vi "4155C Config VAR2 params.vi"(4 "power compliance (0 = OFF)":dbl format="%^.2e", 6 "compliance":dbl=0.1 format="%^.2e", 7 "step":dbl=5.0 format="%^.4e", 8 "error in (no error)":errorcluster, 9 "stop":dbl=10.0 format="%^.4e", 10 "start":dbl format="%^.4e", 11 "VISA session":refnum<visa-resource-name>) -> (0 "error out":errorcluster, 1 "Corrected Step":dbl format="%.2f", 2 "Number of points":i32=1, 3 "dup VISA resource name":refnum<visa-resource-name>)   [LabVIEW 2019]
doc: "This VI configures the secondary sweep source (VAR2) for a sweep mode measurement. \n* This VI does not perform error checking on MEASUREMENT MODE or UNIT TYPE of VAR1, therefore it is the application programmer's responsibility to make certain this VI is used in the proper mode."
panel:
  # "(W)"
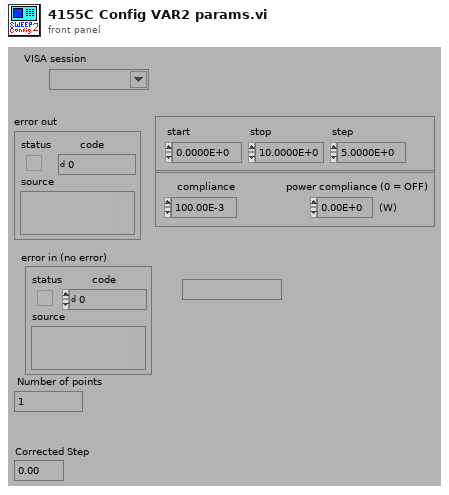
[diagram p1: front panel]
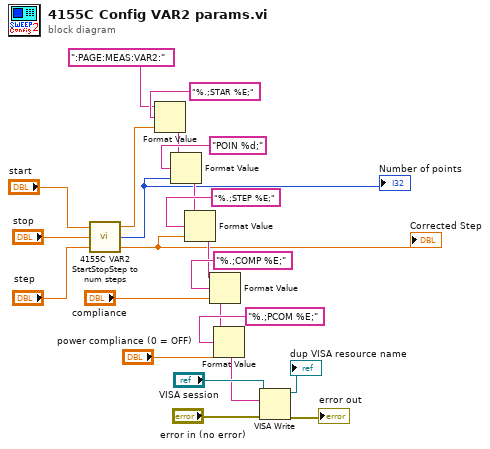
[diagram p0: block diagram]
diagram:
  n1 = call "4155C VAR2 StartStopStep to num steps.vi"("step"="step", "stop"="stop", "start"="start") -> ("Corrected Step"=w1:dbl, "Number of points"=w2:i32, "dup start"=w5:dbl)
  "Number of points" <- w2
  "Corrected Step" <- w1
  n2 = Format Value(string ("")=":PAGE:MEAS:VAR2:", format string="%.;STAR %E;", value (0)=w5) -> (output string=w21:string)
  n3 = Format Value(string ("")=w21, format string="POIN %d;", value (0)=w2) -> (output string=w3:string)
  n4 = Format Value(string ("")=w3, format string="%.;STEP %E;", value (0)=w1) -> (output string=w4:string)
  n5 = Format Value(string ("")=w4, format string="%.;COMP %E;", value (0)="compliance") -> (output string=w17:string)
  n6 = Format Value(string ("")=w17, format string="%.;PCOM %E;", value (0)="power compliance (0 = OFF)") -> (output string=w12:string)
  n7 = VISA Write(VISA resource name="VISA session", write buffer=w12, error in (no error)="error in (no error)") -> (VISA resource name out=→"dup VISA resource name":refnum<visa-resource-name>, error out=→"error out":errorcluster)  [unwired: 1 out]
